vi "Cache-Write.vi"(8 "error in":errorcluster, 10 "Data":T1={"Status"=0, "Ref1"="9998887770", "Serial1"="12345679", "Ref2"="", "Serial2"="", "Values"=[1.0, 2.0, 1.0, 1.0, 1.0, 4.0, 5.0, 1.0]} {"Values" format="%.3f"}, 11 "Idx":i32) -> (0 "error out":errorcluster, 2 "Saved":bool)   [LabVIEW 2016]
doc: "Go to DB->WriteStationValues action\nReturn boolean flag to show if data was saved to DB successfully\n\nWabco 2017 All right reserved\nAuthor: maciej.szupienko@wabco-auto.com"
uses:
  Cache.Action.ctl
  Drivers/PLC/LowLevel/PLC.DataBlock.PLCvalues.ctl
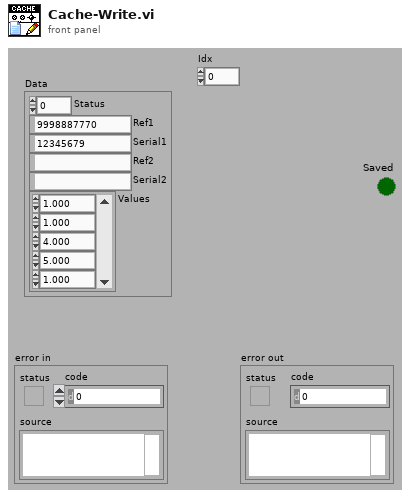
[diagram p1: front panel]
types:
  T1 = typedef "PLC.DataBlock.PLCvalues.ctl" = cluster{"Status":u8, "Ref1":string, "Serial1":string, "Ref2":string, "Serial2":string, "Values":sgl[]}
  T2 = typedef "Cache.Action.ctl" = enum32{"idle", "constructor", "destructor", "--- Cache ---", "Write", "Read", "CheckStatus", "Move", "Delete", "Find"}
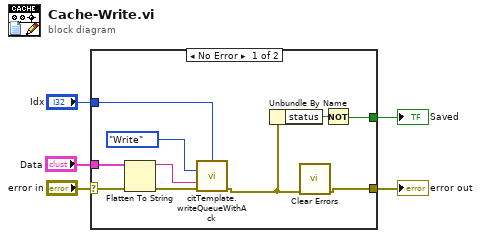
[diagram p0: block diagram]
diagram:
  n1 = case shown="No Error" "error in" {
    selector: "error in" -> [w15 w16]
    tunnel: [w8 w16] -> w4
    tunnel: "Data" -> [w14 _]
    tunnel: "Idx" -> [w10 _]
    tunnel: [w6 _] -> w1
    frame No Error {
      n2 = Flatten To String(anything=w14, error in (no error)=w15) -> (data string=w13:string, error out=w12:errorcluster)  [unwired: 2 in, 1 out]
      n3 = call "citTemplate.writeQueueWithAck.vi"("instance (0)"=w10, "event in"=Cache.Action."Write" ("Action"), "(flatten) data in"=w13, "error in (no error)"=w12) -> ("error out"=w7:errorcluster)  [unwired: 9 in, 2 out]
      n4 = Unbundle By Name(w7) -> ("status"=w9:bool)
      n5 = call <vilib>:"Clear Errors.vi"("error in (no error)"=w7) -> ("error out"=w8:errorcluster)  [unwired: 5 in, 1 out]
      n6 = Not(x=w9) -> (.not. x?=w6:bool)
    }
    frame Error {
    }
  }
  "error out" <- w4
  "Saved" <- w1
